vi "Query Trace Data.vi"(8 "error in (no error)":errorcluster, 10 "Trace Number":u8=1, 11 "VNA-Keysight PNA in":refnum<class "VNA-Keysight PNA.lvclass">) -> (0 "error out":errorcluster, 1 "Data":dbl[](array[numeric]), 2 "Frequency":dbl[](array[numeric]), 3 "VNA-Keysight PNA out":refnum<class "VNA-Keysight PNA.lvclass">)   [LabVIEW 2020, in "VNA-Keysight PNA.lvclass"]
doc: "Query the active trace data.\nIt returns both x and y data"
uses:
  VNA-Keysight PNA.lvclass
  C:/Sandbox/RF Bench/Source Code/WiSpry Test Framework/Instruments/Instrument.lvclass
  C:/Sandbox/RF Bench/Source Code/WiSpry Test Framework/Instruments/Vector Network Analyzer/Vector Network Analyzer.lvclass
  Vector Network Analyzer.lvclass/Vector Network Analyzer.ctl
  Instrument.lvclass/Instrument.ctl
  Instrument.lvclass
  <instrlib>/Keysight PNA Series/Keysight PNA Series.lvlib
  Vector Network Analyzer.lvclass
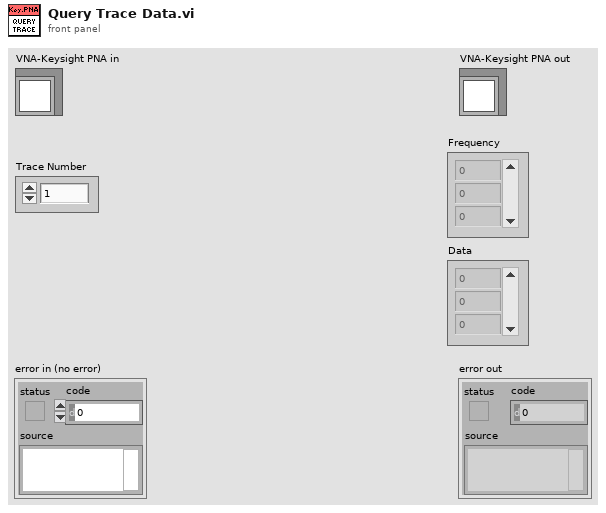
[diagram p1: front panel]
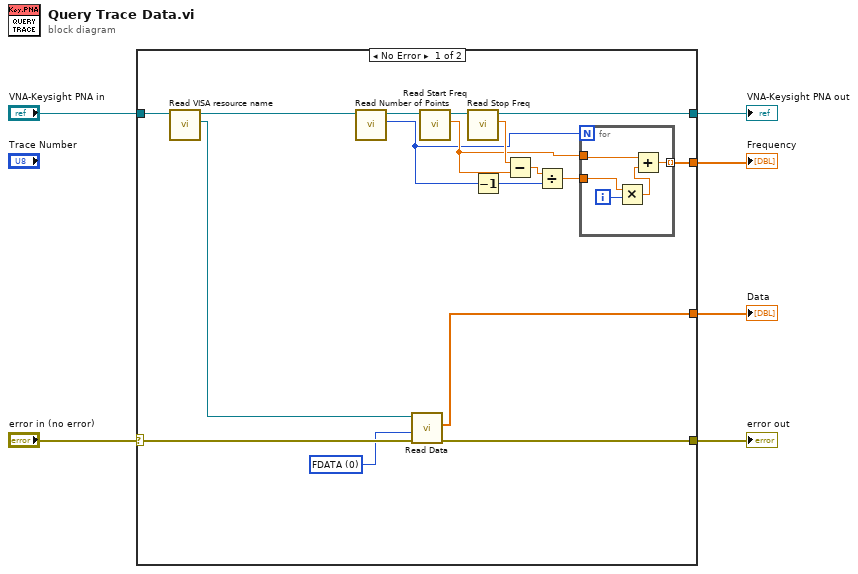
[diagram p0: block diagram]
diagram:
  n1 = case shown="No Error" "error in (no error)" {
    selector: "error in (no error)" -> [w21 w29]
    tunnel: [w9 w30] -> w3
    tunnel: "VNA-Keysight PNA in" -> [w23 w30]
    tunnel: [w7 w29] -> w5
    tunnel: [w19 _] -> w2
    tunnel: [w8 _] -> w1
    frame No Error {
      w20 = 0 items=["FDATA", "RDATA", "SDATA", "FMEM", "SMEM", "SDIV"] ("Data Type (0: FDATA)")
      n2 = call "Read VISA resource name.vi"("Instrument in"=w23) -> ("VISA resource name"=w22:refnum<visa-resource-name>, "Instrument out"=w10:refnum<class "VNA-Keysight PNA.lvclass">)  [unwired: 9 in]
      n3 = call "Read Number of Points.vi"("Vector Network Analyzer in"=w10) -> ("Number of Points"=w11:i32, "Vector Network Analyzer out"=w18:refnum<class "VNA-Keysight PNA.lvclass">)  [unwired: 9 in]
      n4 = call <instrlib>:"Read Data.vi"("error in (no error)"=w21, "Data Type (0: FDATA)"=w20, "VISA resource name"=w22) -> ("error out"=w7:errorcluster, "Data"=w19:dbl[])  [unwired: 6 in, 1 out]
      n5 = call "Read Start Freq.vi"("Vector Network Analyzer in"=w18) -> ("Start Freq"=w14:dbl, "Vector Network Analyzer out"=w17:refnum<class "VNA-Keysight PNA.lvclass">)  [unwired: 9 in]
      n6 = call "Read Stop Freq.vi"("Vector Network Analyzer in"=w17) -> ("Stop Freq"=w16:dbl, "Vector Network Analyzer out"=w9:refnum<class "VNA-Keysight PNA.lvclass">)  [unwired: 9 in]
      n7 = Decrement(x=w11) -> (x-1=w12:i32)
      n8 = Subtract(x=w16, y=w14) -> (x-y=w15:dbl)
      n9 = Divide(x=w15, y=w12) -> (x/y=w13:dbl)
      n10 = for {
        N: w11 -> [_]
        tunnel: w14 -> [w25]
        tunnel: w13 -> [w27]
        tunnel: [w24] -> w8 mode=indexing
        i -> [w28]
        n11 = Multiply(x=w27, y=w28) -> (x*y=w26:dbl)
        n12 = Add(x=w25, y=w26) -> (x+y=w24:dbl)
      }
    }
    frame Error {
    }
  }
  "error out" <- w5
  "VNA-Keysight PNA out" <- w3
  "Data" <- w2
  "Frequency" <- w1
